vi "FPGA_TimedLoopTest2.vi"() -> ()   [LabVIEW 2014]
uses:
  <vilib>/Platform/TimedLoop/XDataNode/timing_clust.ctl
  <vilib>/Platform/TimedLoop/XDataNode/nitl_modes.ctl
  <vilib>/Platform/TimedLoop/XDataNode/wakeup.ctl
  <vilib>/rvi/Emulation/niFpgaSctlEmulationGetInTimedLoop.vi
  <vilib>/rvi/Emulation/niFpgaEmulationReportErrorSimple.vi
  <vilib>/rvi/Emulation/niFpgaGetClockAttributes.vi
  <vilib>/rvi/Emulation/niFpgaCriticalErrorInLSC.vi
  <vilib>/platform/TimedLoop/XDataNode/XDataNode.xnode
  <vilib>/rvi/FXPMathLib/FxpMul/XNode/nifxpmath_Multiplier.xnode
  <vilib>/Platform/TimedLoop/XDataNode/XDNodeRunTimeDep.lvlib
  <vilib>/rvi/FXPMathLib/sim/FxpSim.dll
panel:
  out "x*y":fxp<+,6,4>
  out "TimeDelta":u32
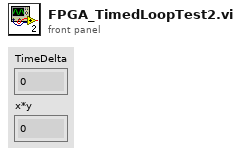
[diagram p1: front panel]
types:
  T1 = typedef "XDNodeRunTimeDep.lvlib/timing_clust.ctl" = cluster{"Expected End [f-1]":u64, "Actual End [f-1]":u64, "Finished Late? [f-1]":bool, "Expected End [i-1]":u64, "Actual End [i-1]":u64, "Finished Late? [i-1]":bool, "Expected Start [i]":u64, "Actual Start [i]":u64, "Expected Start [f]":u64, "Actual Start [f]":u64, "Source Name":string, "Structure Name":string, "Period":i64, "Deadline":i64, "Offset":i64, "Start":i64, "Priority":i32, "Timeout":i32, "Mode":T2, "Wakeup Reason":T3, "Error":errorcluster, "Source Type":string, "Secondary Source Type":string, "Global End Time":u64, "Global Start Time":u64, "Frame Duration":u64, "Iteration Duration":u64, "Assigned CPU":i32, "I/O Scan Engine Mode":u32}
  T2 = typedef "XDNodeRunTimeDep.lvlib/nitl_modes.ctl" = enum32{"No Change", "Process missed periods, maintain original phase", "Discard missed periods, maintain original phase", "Process missed periods, ignore original phase", "Discard missed periods, ignore original phase"}
  T3 = typedef "XDNodeRunTimeDep.lvlib/wakeup.ctl" = enum32{"Normal", "Aborted", "Asynchronous wakeup", "Timing source error", "Timed loop error", "Timeout"}
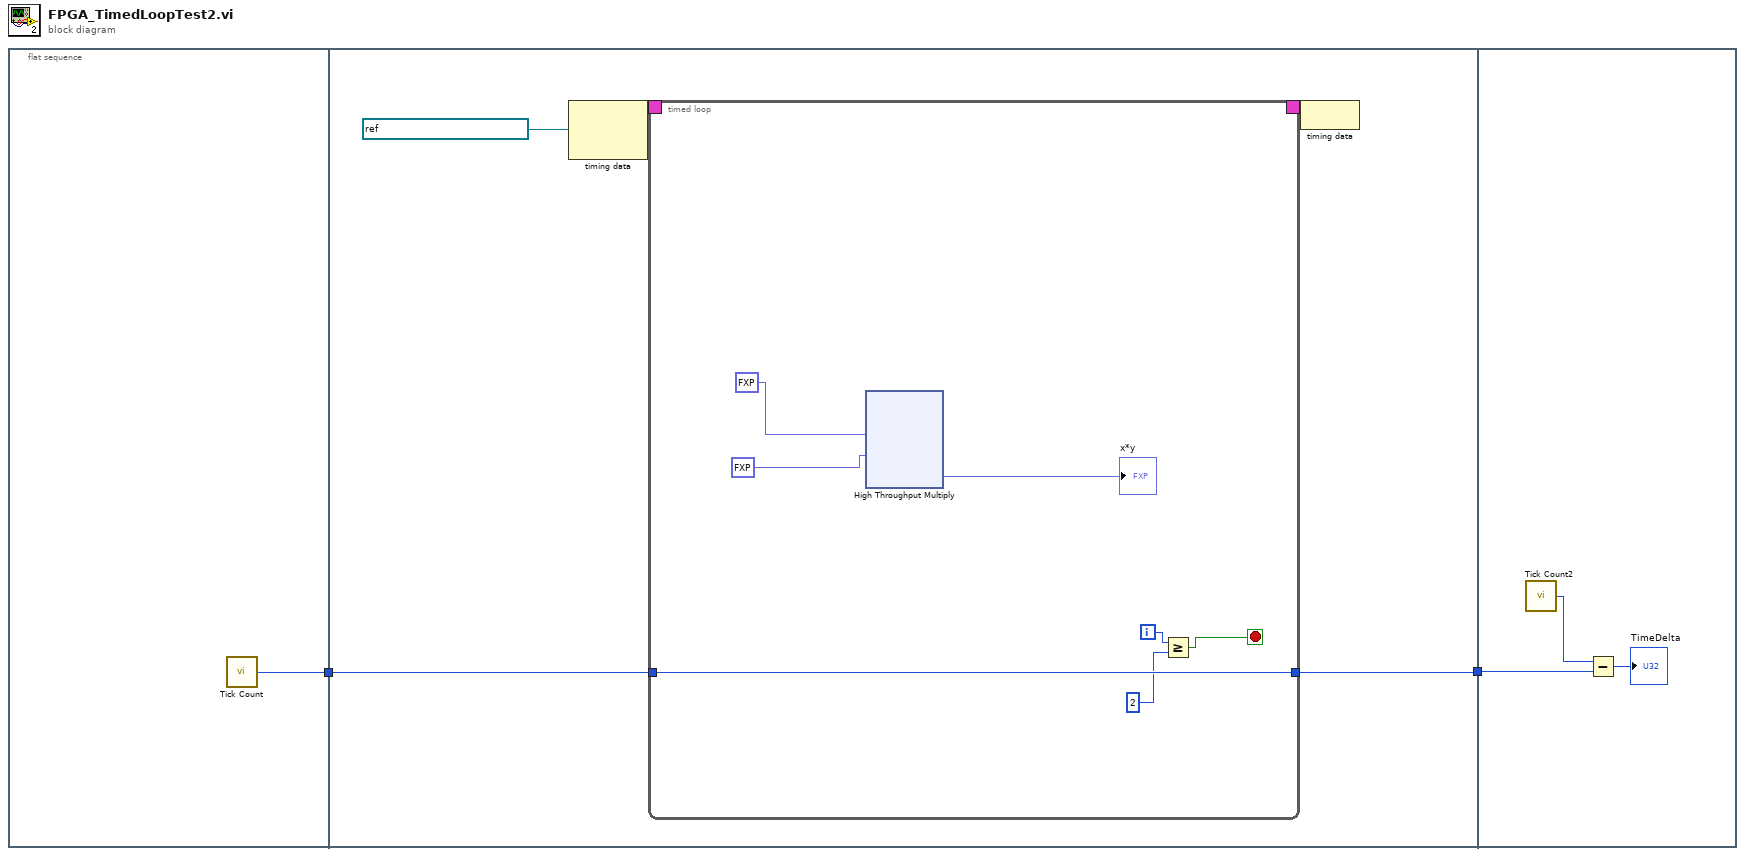
[diagram p0: block diagram]
diagram:
  n1 = flat-sequence {
    tunnel: [w3] -> w2
    tunnel: w2 -> [w5]
    tunnel: [w4] -> w1
    tunnel: w1 -> [w23]
    frame #0 {
      n2 = call "Tick Count"() -> ("Tick Count(mSec)"=w3:u32)
    }
    frame #1 {
      n3 = node-c288(refnum<k21> "40 MHz Onboard Clock" ("Source Name")) -> (w8:T1)  [unwired: 1 in]
      n4 = timed-loop {
        timing: w8 -> [_]
        timing-out: [_] -> w7
        tunnel: w5 -> [w15]
        tunnel: [w15] -> w4
        i -> [w14]
        stop <- w12 stop-if-true
        n5 = xnode ("High Throughput Multiply")("x"=fxp<+,3,2> 2.5, "y"=fxp<+,3,2> 2.5) -> ("x*y"=→"x*y":fxp<+,6,4>)
        n6 = Greater Or Equal?(x=w14, y=2) -> (x >= y?=w12:bool)
      }
      n7 = node-c288(w7) -> ()
    }
    frame #2 {
      n8 = call "Tick Count2"() -> ("Tick Count(mSec)"=w24:u32)
      n9 = Subtract(x=w24, y=w23) -> (x-y=→"TimeDelta":u32)
    }
  }
